vi "Get PID Configuration.vi"(8 "error in (no error)":errorcluster, 11 "connection info":T3) -> (0 "error out":errorcluster, 1 "Timed Out?":bool, 2 "Settings":T1, 3 "connection info":T3)   [LabVIEW 2019, in "Control Host Automation API.lvlib"]
uses:
  Control Host Automation API.lvlib
  Addon/Addon Shared/Types/Gain Schedule.ctl
  Addon/Addon Shared/Control Addon Shared.lvlib
  Addon/Addon Shared/Types/Get Settings Message.ctl
  <vilib>/NI/NI VeriStand Addon Network Comm/Shared/NI VeriStand Addon Network Comm Shared.lvlib
  <vilib>/NI/STM/SubVIs/MetaDataElement.ctl
  <vilib>/NI/STM/NI STM.lvlib
  <vilib>/NI/STM/TCP/TCP Connection Info.ctl
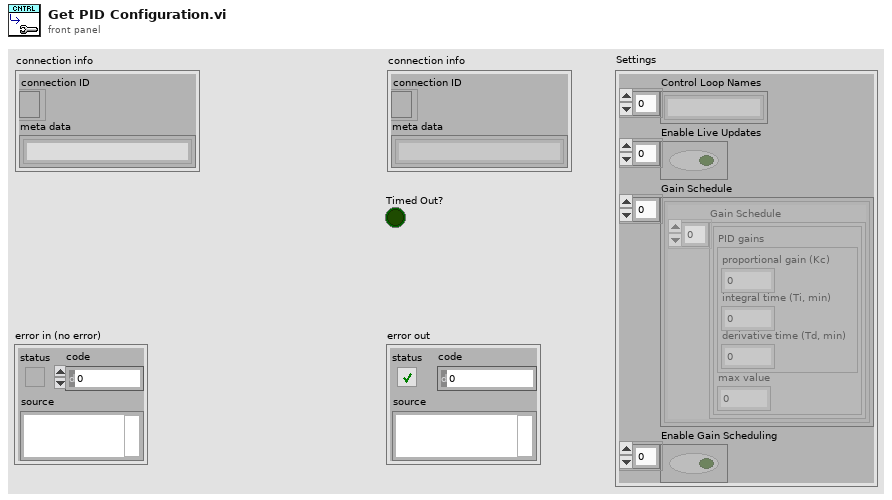
[diagram p1: front panel]
types:
  T1 = typedef "Control Addon Shared.lvlib/Get Settings Message.ctl" = cluster{"Control Loop Names":string[], "Enable Live Updates":bool[], "Gain Schedule":T2[], "Enable Gain Scheduling":bool[]}
  T2 = typedef "Control Addon Shared.lvlib/Gain Schedule.ctl" = cluster{"Gain Schedule":cluster{"PID gains":cluster{"proportional gain (Kc)":dbl, "integral time (Ti, min)":dbl, "derivative time (Td, min)":dbl}, "max value":dbl}[]}
  T3 = typedef "NI STM.lvlib/TCP Connection Info.ctl" = cluster{"connection ID":refnum<k5>, "meta data":T4[]}
  T4 = typedef "NI STM.lvlib/MetaDataElement.ctl" = string
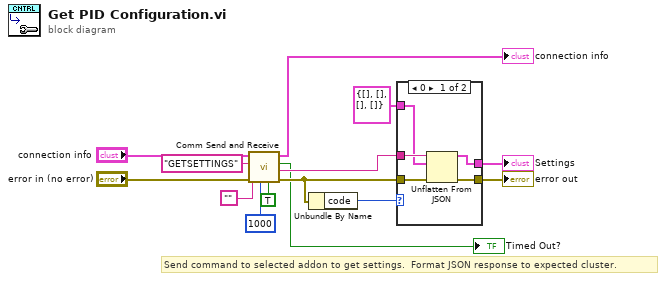
[diagram p0: block diagram]
diagram:
  # "Send command to selected addon to get settings.  Format JSON response to expected cluster."
  n1 = call <vilib>:"Comm Send and Receive.vi"("Resp Required?"=TRUE, "Timeout (ms)"=u32 1000 ("Timeout ms (5000)"), "error in (no error)"="error in (no error)", "Data"="", "Name"="GETSETTINGS", "connection info"="connection info") -> ("error out"=w7:errorcluster, "Data"=w10:string, "Timed Out?"=→"Timed Out?":bool, "connection info"=→"connection info":T3)  [unwired: 2 in]
  n2 = Unbundle By Name(w7) -> ("code"=w6:i32)
  n3 = case shown="0" w6 {
    tunnel: w10 -> [w19 _]
    tunnel: w7 -> [w18 w21]
    tunnel: [w17 w21] -> w9
    tunnel: [w16 w20] -> w8
    tunnel: T1 {"Control Loop Names"=[], "Enable Live Updates"=[], "Gain Schedule"=[], "Enable Gain Scheduling"=[]} ("GetSettings") -> [w15 w20]
    frame 0 {
      n4 = Unflatten From JSON(JSON string=w19, type and defaults=w15, error in (no error)=w18) -> (value=w16:T1, error out=w17:errorcluster)  [unwired: 4 in]
    }
    frame Default {
    }
  }
  "error out" <- w9
  "Settings" <- w8
